vi "DSF.Memory.Cache.Framework.Set Plugin Caches.vi"(8 "error in (no error)":errorcluster, 10 "Plugin Caches":refnum<class "DSF.Memory.Cache.Plugin.lvclass">[](array[class]), 11 "Framework Cache in":refnum<class "DSF.Memory.Cache.Framework.lvclass">) -> (0 "error out":errorcluster, 3 "Framework Cache out":refnum<class "DSF.Memory.Cache.Framework.lvclass">)   [LabVIEW 2016, in "DSF.Memory.lvlib" / "DSF.Memory.Cache.Framework.lvclass"]
uses:
  DSF.Memory.Cache.Framework.lvclass
  DSF.Memory.Cache.Plugin.lvclass
  DSF.Memory.Cache.Framework.lvclass/DSF.Memory.Cache.Framework.ctl
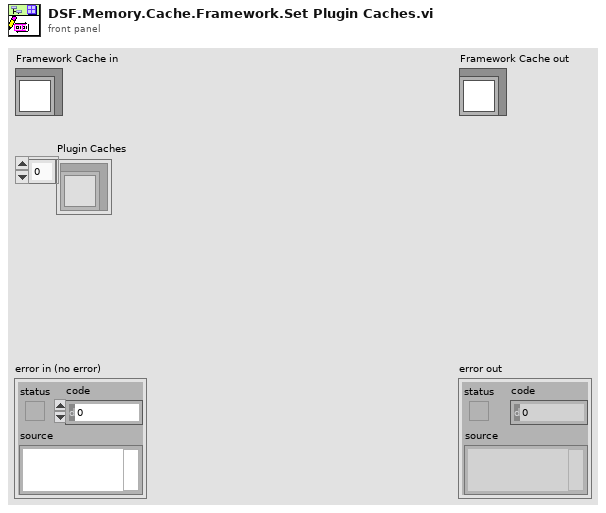
[diagram p1: front panel]
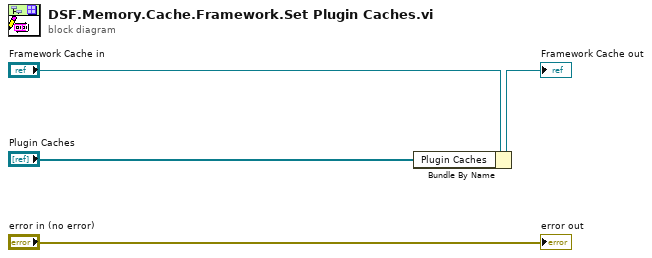
[diagram p0: block diagram]
diagram:
  n1 = Bundle By Name(cluster="Framework Cache in", "Plugin Caches"="Plugin Caches") -> (→"Framework Cache out":refnum<class "DSF.Memory.Cache.Framework.lvclass">)
  "error out" <- "error in (no error)"
